vi "GetSignalParams.vi"(8 "error in (no error)":errorcluster, 11 "PmuTestFunctions in":refnum<class "PmuTestFunctions.lvclass">) -> (0 "error out":errorcluster, 2 "FitterParams":variant, 3 "PmuTestFunctions out":refnum<class "PmuTestFunctions.lvclass">)   [LabVIEW 2014, in "Functions.lvlib" / "PmuTestFunctions.lvclass"]
uses:
  PmuTestFunctions.lvclass
  PmuTestFunctions.lvclass/PmuTestFunctions.ctl
  Accessors/Read PmuTestParams.vi
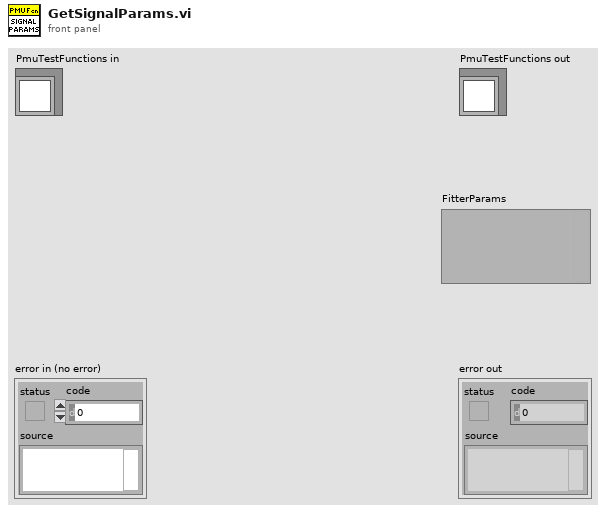
[diagram p1: front panel]
types:
  T1 = typedef "Functions.lvlib/PmuTestFunctions.lvclass/PmuTestParams.ctl" = dbl[][]
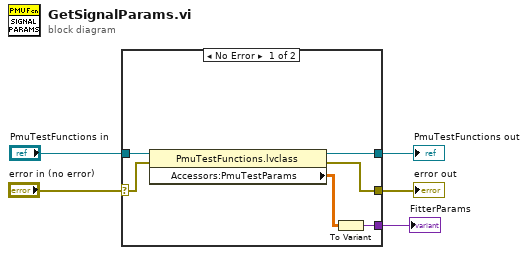
[diagram p0: block diagram]
diagram:
  n1 = case shown="No Error" "error in (no error)" {
    selector: "error in (no error)" -> [w10 w13]
    tunnel: [w8 w13] -> w4
    tunnel: "PmuTestFunctions in" -> [w11 w12]
    tunnel: [w9 w12] -> w2
    tunnel: [w6 _] -> w1
    frame No Error {
      n2 = property class="PmuTestFunctions.lvclass"(reference=w11, error in=w10) -> (reference out=w9:refnum<class "PmuTestFunctions.lvclass">, error out=w8:errorcluster, "Accessors:PmuTestParams"=w7:T1)
      n3 = To Variant(anything=w7) -> (Variant=w6:variant)
    }
    frame Error {
    }
  }
  "error out" <- w4
  "PmuTestFunctions out" <- w2
  "FitterParams" <- w1
